vi "Load.vi"(8 "Error In":errorcluster, 10 "Key":string, 11 "Loader In":refnum<class "Data.lvclass">) -> (0 "Error Out":errorcluster, 2 "Template":string, 3 "Loader Out":refnum<class "Data.lvclass">)   [LabVIEW 2018, in "Toolkit.lvlib" / "Loaders.lvlib" / "Data.lvclass"]
doc: "Gets a template as a string based on the Partial's key value in the root, or master, template."
uses:
  Data.lvclass
  Data.lvclass/Data.ctl
  Data/Path/Path.lvclass
  Data/Path/Path.lvclass/Path.ctl
  Data/String/String.lvclass
  Data/String/String.lvclass/String.ctl
  Data/Datum/Datum.lvclass
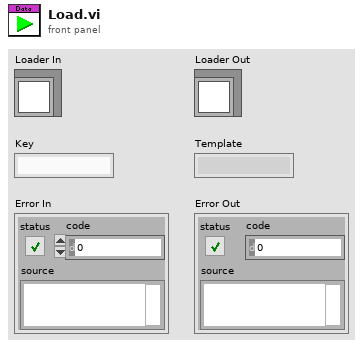
[diagram p1: front panel]
types:
  T1 = enum16{"open", "replace", "create", "open or create", "replace or create", "replace or create with confirmation"}
  T2 = cluster{"Key":string, "Value":refnum<class "Datum.lvclass">}[]
  T3 = typedef "Toolkit.lvlib/Data.lvlib/Types.ctl" = enum16{"Array", "Boolean", "Function", "Map", "Null", "Path", "String", "Unknown"}
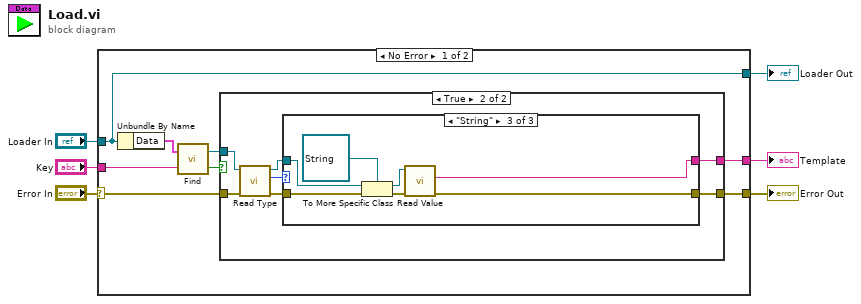
[diagram p0: block diagram]
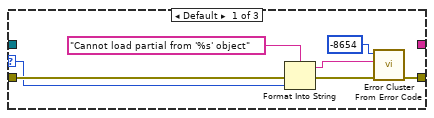
[diagram p3: hidden frame]
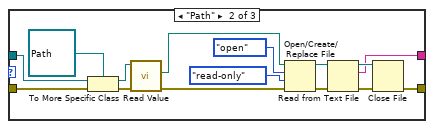
[diagram p4: hidden frame]
diagram:
  n1 = case shown="No Error" "Error In" {
    selector: "Error In" -> [w7 w53]
    tunnel: "Loader In" -> [w9 w52]
    tunnel: "Key" -> [w14 _]
    tunnel: [w10 w53] -> w3
    tunnel: [w9 w52] -> w2
    tunnel: [w11 _] -> w1
    frame No Error {
      n2 = Unbundle By Name(w9) -> ("Data"=w8:T2)
      n3 = call "Find.vi"("Key"=w14, "Data"=w8) -> ("Found?"=w13:bool, "Value"=w12:refnum<class "Datum.lvclass">)
      n4 = case shown="True" w13 {
        tunnel: w7 -> [w15 w18]
        tunnel: w12 -> [_ w22]
        tunnel: [w15 w21] -> w10
        tunnel: [_ w20] -> w11
        frame False {
        }
        frame True {
          n5 = call-dynamic "Read Type.vi"("Error In"=w18, "Datum In"=w22) -> ("Error Out"=w17:errorcluster, "Type"=w16:T3, "Datum Out"=w19:refnum<class "Datum.lvclass">)  [unwired: 7 in]
          n6 = case shown="\"String\"" w16 {
            selector: w16 -> [w25 _ _]
            tunnel: w17 -> [w29 w44 w51]
            tunnel: w19 -> [_ w43 w50]
            tunnel: [w28 w31 w47] -> w21
            tunnel: [_ w30 w45] -> w20
            frame Default {
              n7 = Format Into String(format string="Cannot load partial from '%s' object" ("error message (\"\")"), error in=w29, w25) -> (resulting string=w23:string, error out=w26:errorcluster)  [unwired: 1 in]
              n8 = call <vilib>:"Error Cluster From Error Code.vi"("error in (no error)"=w26, "error message (\"\")"=w23, "error code (0)"=-8654) -> ("error out"=w28:errorcluster)  [unwired: 6 in]
            }
            frame "Path" {
              n9 = To More Specific Class(target class=refnum<class "Path.lvclass"> refnum ("Toolkit.lvlib:Data.lvlib:Path.lvclass"), reference=w43, error in=w44) -> (specific class reference=w40:refnum<class "Path.lvclass">, error out=w41:errorcluster)
              n10 = call "Read Value.vi"("Error In"=w41, "Path In"=w40) -> ("Error Out"=w39:errorcluster, "Value"=w38:path)  [unwired: 7 in, 1 out]
              n11 = Open/Create/Replace File(file path (use dialog)=w38, error in=w39, operation (0:open)=T1."open", access (0:read/write)=enum16{"read/write", "read-only", "write-only"}."read-only") -> (refnum out=w35:refnum<file>, error out=w34:errorcluster)  [unwired: 2 in, 1 out]
              n12 = Read from Text File(file (use dialog)=w35, error in=w34) -> (refnum out=w33:refnum<file>, text=w30:string, error out=w32:errorcluster)  [unwired: 2 in, 1 out]
              n13 = Close File(refnum=w33, error in=w32) -> (error out=w31:errorcluster)  [unwired: 1 out]
            }
            frame "String" {
              n14 = To More Specific Class(target class=refnum<class "String.lvclass"> refnum ("Toolkit.lvlib:Data.lvlib:String.lvclass"), reference=w50, error in=w51) -> (specific class reference=w46:refnum<class "String.lvclass">, error out=w48:errorcluster)
              n15 = call "Read Value.vi"("Error In"=w48, "String In"=w46) -> ("Error Out"=w47:errorcluster, "Value"=w45:string)  [unwired: 7 in, 1 out]
            }
          }
        }
      }
    }
    frame Error {
    }
  }
  "Loader Out" <- w2
  "Error Out" <- w3
  "Template" <- w1
